vi "Set Velocity.vi"(8 "error in (no error)":errorcluster, 10 "velocity":i16, 11 "DC Brick in":refnum<class "DC Brick.lvclass">) -> (0 "error out":errorcluster, 3 "DC Brick out":refnum<class "DC Brick.lvclass">)   [LabVIEW 2011, in "Tinkerforge.lvlib" / "DC Brick.lvclass"]
doc: "This VI sets the velocity of the motor. Whereas -32767 is full speed backward, 0 is stop and 32767 is full speed forward. Depending on the acceleration (see set_acceleration), the motor is not immediately brought to the velocity but smoothly accelerated.\n\nThe velocity describes the duty cycle of the PWM with which the motor is controlled, e.g. a velocity of 3277 sets a PWM with a 10% duty cycle. You can not only control the duty cycle of the PWM but also the frequency, see set_pwm_frequency.\n\nThe default velocity is 0."
uses:
  DC Brick.lvclass
  Device/Device.lvclass
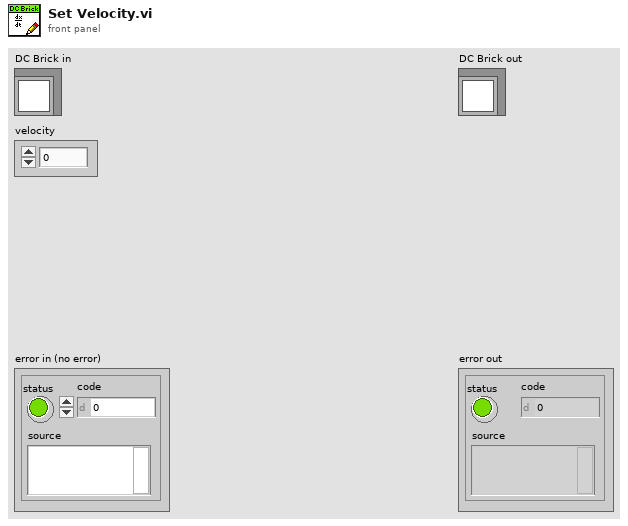
[diagram p1: front panel]
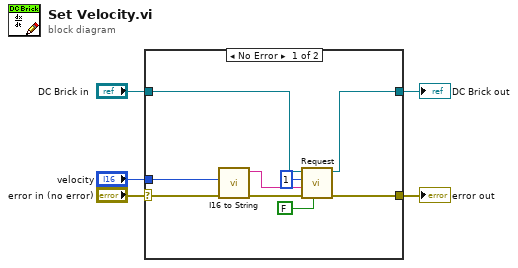
[diagram p0: block diagram]
diagram:
  n1 = case shown="No Error" "error in (no error)" {
    selector: "error in (no error)" -> [w9 w16]
    tunnel: [w10 w16] -> w4
    tunnel: [w13 w15] -> w2
    tunnel: "DC Brick in" -> [w14 w15]
    tunnel: "velocity" -> [w7 _]
    frame No Error {
      n2 = call "I16 to String.vi"("Error In"=w9, "I16"=w7) -> ("Error Out"=w8:errorcluster, "String out"=w6:string)  [unwired: 8 in]
      n3 = call "Request.vi"("Response"=FALSE, "error in (no error)"=w8, "Data"=w6, "Function ID"=u8 1, "Device in"=w14) -> ("error out"=w10:errorcluster, "Device out"=w13:refnum<class "DC Brick.lvclass">)  [unwired: 2 in, 3 out]
    }
    frame Error {
    }
  }
  "error out" <- w4
  "DC Brick out" <- w2
